vi "Dot Product.vi"(10 "Vector B":T1, 11 "Vector A":T1) -> (3 "Dot Product":sgl)   [LabVIEW 2022 SP3, in "3D.lvlib"]
uses:
  3D.lvlib
  Vector 3D.ctl
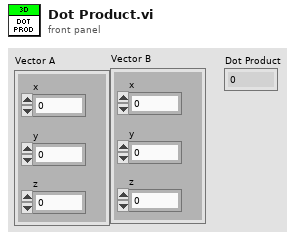
[diagram p1: front panel]
types:
  T1 = typedef "3D.lvlib/Vector 3D.ctl" = cluster{"x":sgl, "y":sgl, "z":sgl}
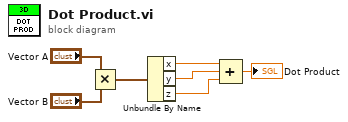
[diagram p0: block diagram]
diagram:
  n1 = Multiply(x="Vector A", y="Vector B") -> (x*y=w5:T1)
  n2 = Unbundle By Name(w5) -> ("x"=w4:sgl, "y"=w3:sgl, "z"=w2:sgl)
  n3 = Compound Arithmetic op=ADD(w4, w3, w2) -> (→"Dot Product":sgl)
